vi "JoinGame.vi"(8 "error in (no error)":errorcluster, 10 "PlayerName":string, 11 "CS++GoBangServer in":refnum<class "CS++GoBangServer.lvclass">) -> (0 "error out":errorcluster, 3 "CS++GoBangServer out":refnum<class "CS++GoBangServer.lvclass">)   [LabVIEW 2013, in "GoBang.lvlib" / "CS++GoBangServer.lvclass"]
uses:
  CS++GoBangServer.lvclass
  Core/Classes/CS++ProcessVariables/ProcessVariable/PV.lvclass
  typdefs/GameState.ctl
  CS++GoBangServer.lvclass/CS++GoBangServer.ctl
  Core/Classes/CS++ProcessVariables/PVConnection/PVConnection.lvclass
  Core/Classes/CS++ProcessVariables/ProcessVariable/PV.lvclass/PV.ctl
  Core/Classes/CS++ProcessVariables/ProcessVariable/Write Data.vi
  Core/Classes/CS++ProcessVariables/ProcessVariable/Write Timestamp.vi
  Core/Classes/CS++ProcessVariables/ProcessVariable/Write Quality.vi
  Core/Classes/CS++ProcessVariables/ProcessVariable/Write status.vi
  GoBang.lvlib
panel:
  in  "Color(True=White)":bool
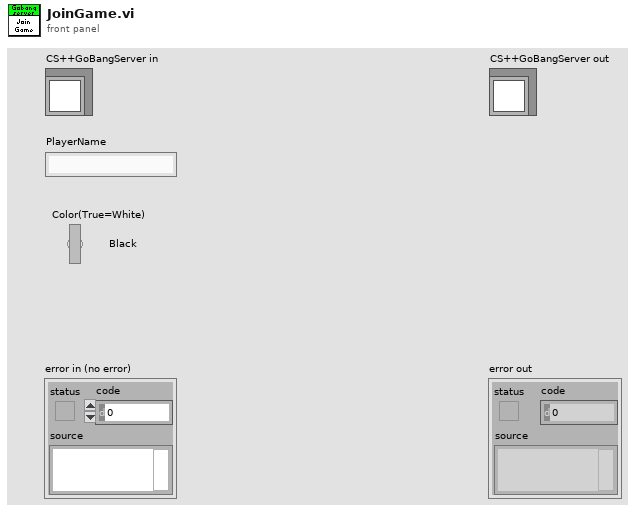
[diagram p1: front panel]
types:
  T1 = typedef "GoBang.lvlib/GameState.ctl" = enum16{"Waiting for opponent", "White to move", "Black to move", "Game over, white won", "Game over, black won"}
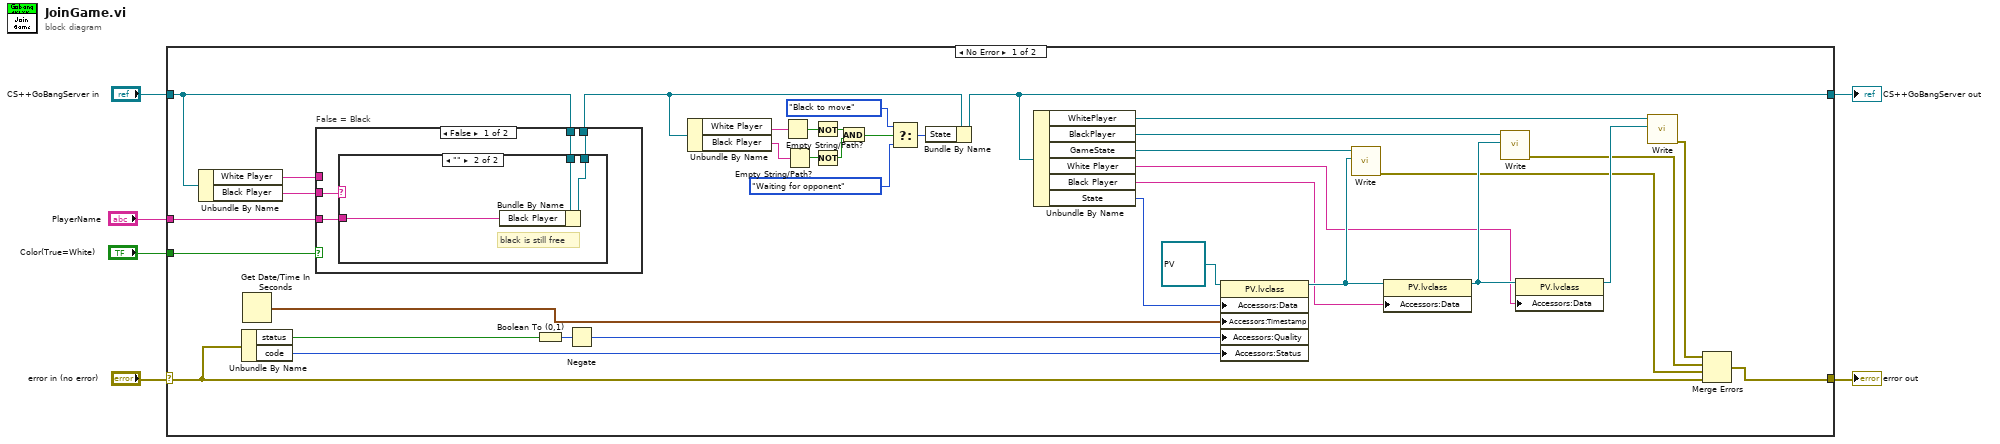
[diagram p0: block diagram]
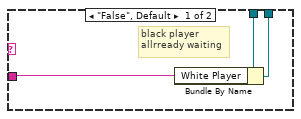
[diagram p2: hidden frame]
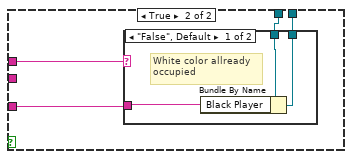
[diagram p3: hidden frame]
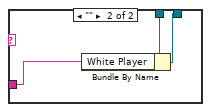
[diagram p4: hidden frame]
diagram:
  n1 = case shown="No Error" "error in (no error)" {
    selector: "error in (no error)" -> [w30 w65]
    tunnel: [w22 w65] -> w5
    tunnel: [w8 w64] -> w3
    tunnel: "CS++GoBangServer in" -> [w41 w64]
    tunnel: "Color(True=White)" -> [w43 _]
    tunnel: "PlayerName" -> [w40 _]
    frame No Error {
      n2 = Unbundle By Name(w41) -> ("White Player"=w39:string, "Black Player"=w42:string)
      n3 = Unbundle By Name(w30) -> ("status"=w35:bool, "code"=w29:i32)
      n4 = Get Date/Time In Seconds() -> (seconds since 1Jan1904=w33:timestamp)
      n5 = case "False = Black" shown="False" w43 {
        tunnel: w42 -> [w45 _]
        tunnel: w41 -> [w47 w57]
        tunnel: [w46 w56] -> w18
        tunnel: w40 -> [w44 w55]
        tunnel: w39 -> [_ w54]
        frame False {
          n6 = case shown="\"\"" w45 {
            tunnel: w47 -> [w49 w53]
            tunnel: [w50 w52] -> w46
            tunnel: w44 -> [w48 w51]
            frame "False", Default {
              # "black player\nallrready waiting"
              n7 = Bundle By Name(cluster=w49, "White Player"=w48) -> (w50:refnum<class "CS++GoBangServer.lvclass">)
            }
            frame "" {
              # "black is still free"
              n8 = Bundle By Name(cluster=w53, "Black Player"=w51) -> (w52:refnum<class "CS++GoBangServer.lvclass">)
            }
          }
        }
        frame True {
          n9 = case shown="\"False\", Default" w54 {
            tunnel: w57 -> [w59 w63]
            tunnel: [w60 w62] -> w56
            tunnel: w55 -> [w58 w61]
            frame "False", Default {
              # "White color allready \noccupied"
              n10 = Bundle By Name(cluster=w59, "Black Player"=w58) -> (w60:refnum<class "CS++GoBangServer.lvclass">)
            }
            frame "" {
              n11 = Bundle By Name(cluster=w63, "White Player"=w61) -> (w62:refnum<class "CS++GoBangServer.lvclass">)
            }
          }
        }
      }
      n12 = Boolean To (0,1)(Boolean=w35) -> (0, 1=w34:i16)
      n13 = Negate(x=w34) -> (-x=w31:i16)
      n14 = Unbundle By Name(w18) -> ("White Player"=w17:string, "Black Player"=w16:string)
      n15 = Empty String/Path?(string/path=w17) -> (empty?=w14:bool)
      n16 = Empty String/Path?(string/path=w16) -> (empty?=w15:bool)
      n17 = Not(x=w14) -> (.not. x?=w13:bool)
      n18 = Not(x=w15) -> (.not. x?=w12:bool)
      n19 = And(x=w13, y=w12) -> (x .and. y?=w11:bool)
      n20 = Select(t=GameState."Black to move" ("State"), s=w11, f=GameState."Waiting for opponent" ("State")) -> (s? t:f=w7:T1)
      n21 = Bundle By Name(cluster=w18, "State"=w7) -> (w8:refnum<class "CS++GoBangServer.lvclass">)
      n22 = Unbundle By Name(w8) -> ("WhitePlayer"=w38:refnum<class "PVConnection.lvclass">, "BlackPlayer"=w36:refnum<class "PVConnection.lvclass">, "GameState"=w37:refnum<class "PVConnection.lvclass">, "White Player"=w24:string, "Black Player"=w26:string, "State"=w32:T1)
      n23 = property class="PV.lvclass"(reference=refnum<class "PV.lvclass"> refnum ("CS++ProcessVariables.lvlib:PV.lvclass"), "Accessors:Data"=w32, "Accessors:Timestamp"=w33, "Accessors:Quality"=w31, "Accessors:Status"=w29) -> (reference out=w27:refnum<class "PV.lvclass">)  [unwired: 1 in, 1 out]
      n24 = call-dynamic "Write.vi"("PV"=w27, "PVConnection in"=w37) -> ("error out"=w19:errorcluster)  [unwired: 8 in, 1 out]
      n25 = property class="PV.lvclass"(reference=w27, "Accessors:Data"=w26) -> (reference out=w25:refnum<class "PV.lvclass">)  [unwired: 1 in, 1 out]
      n26 = call-dynamic "Write.vi"("PV"=w25, "PVConnection in"=w36) -> ("error out"=w20:errorcluster)  [unwired: 8 in, 1 out]
      n27 = property class="PV.lvclass"(reference=w25, "Accessors:Data"=w24) -> (reference out=w23:refnum<class "PV.lvclass">)  [unwired: 1 in, 1 out]
      n28 = call-dynamic "Write.vi"("PV"=w23, "PVConnection in"=w38) -> ("error out"=w21:errorcluster)  [unwired: 8 in, 1 out]
      n29 = Merge Errors(w21, w20, w19, w30) -> (w22:errorcluster)
    }
    frame Error {
    }
  }
  "error out" <- w5
  "CS++GoBangServer out" <- w3
